vi "Read ADU Packet1.vi"(8 "error in":errorcluster, 10 "isMaster (f)":bool, 11 "RTU transmission data unit in":refnum<class "RTU Data Unit.lvclass">) -> (0 "error out":errorcluster, 1 "modbus data unit":refnum<class "Modbus Data Unit.lvclass">, 3 "RTU transmission data unit out":refnum<class "RTU Data Unit.lvclass">, 5 "PDU Valid?":bool)   [LabVIEW 2021, in "RTU Data Unit.lvclass"]
doc: "This uses the protocol layer to read a modbus packet off of the bus, wrapped in the RTU transmission data unit."
uses:
  RTU Data Unit.lvclass
  D:/my_projects/projects/Algorithms/Labview/21/Modbus_v121c/Transmission Data Unit/Serial Interface/Serial Data Unit.lvclass
  D:/my_projects/projects/Algorithms/Labview/21/Modbus_v121c/Transmission Data Unit/Transmission Data Unit.lvclass
  Modbus Data Unit/Modbus Data Unit.lvclass
  Transmission Data Unit.lvclass/Transmission Data Unit.ctl
  Serial Interface/Serial Data Unit.lvclass/Serial Data Unit.ctl
  Modbus Data Unit/Modbus Data Unit.lvclass/Modbus Data Unit.ctl
  <vilib>/ErrorRing/Error Ring.xnode
  Serial Interface/Serial Data Unit.lvclass
  Transmission Data Unit.lvclass
  Network Interface/Serial Interface/Serial Shared Components/Serial Shared Components.lvlib
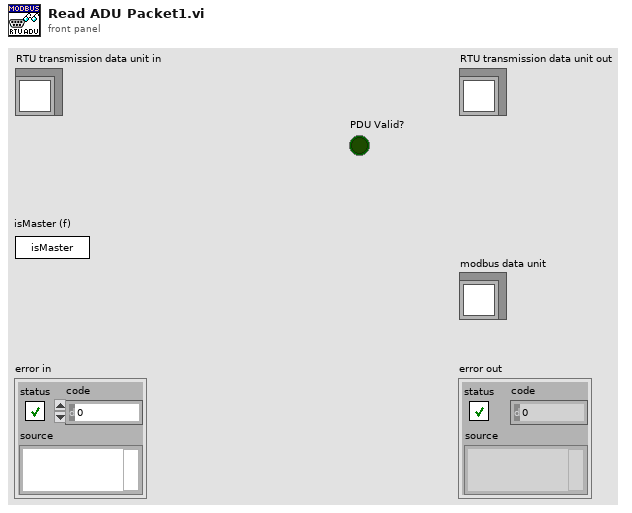
[diagram p1: front panel]
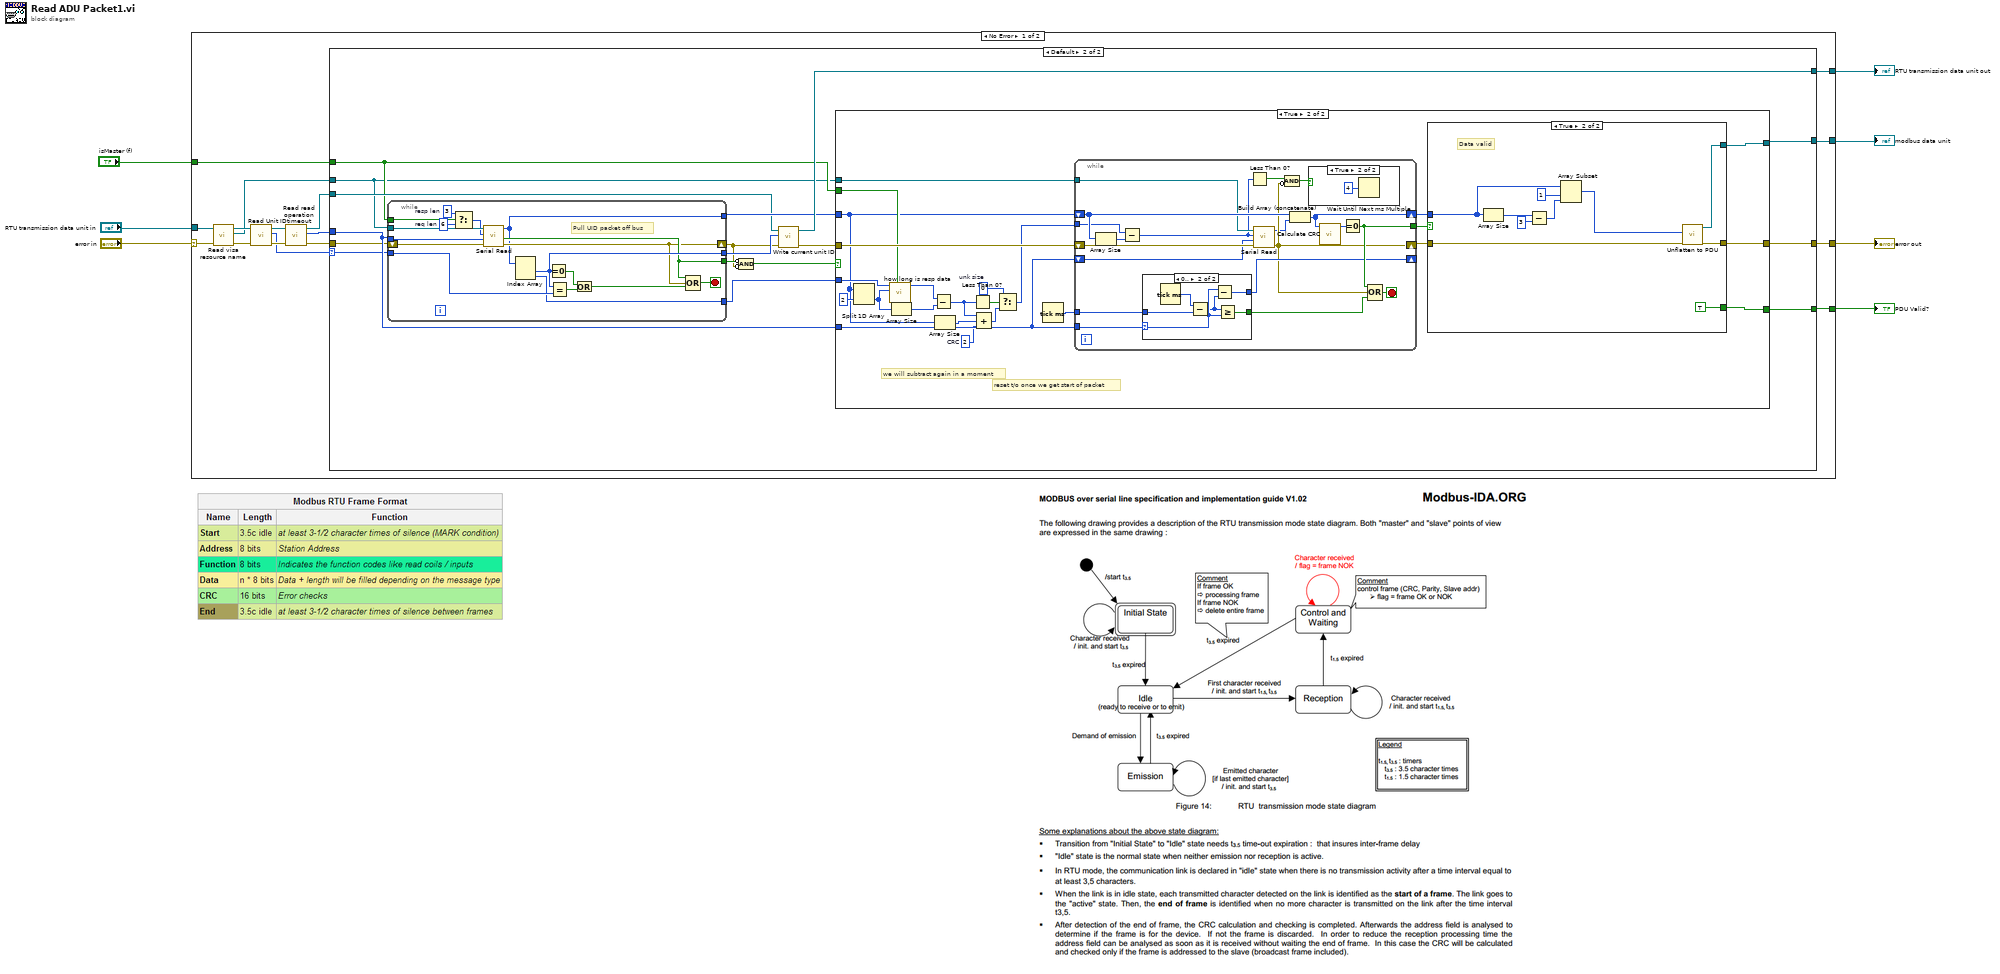
[diagram p0: block diagram]
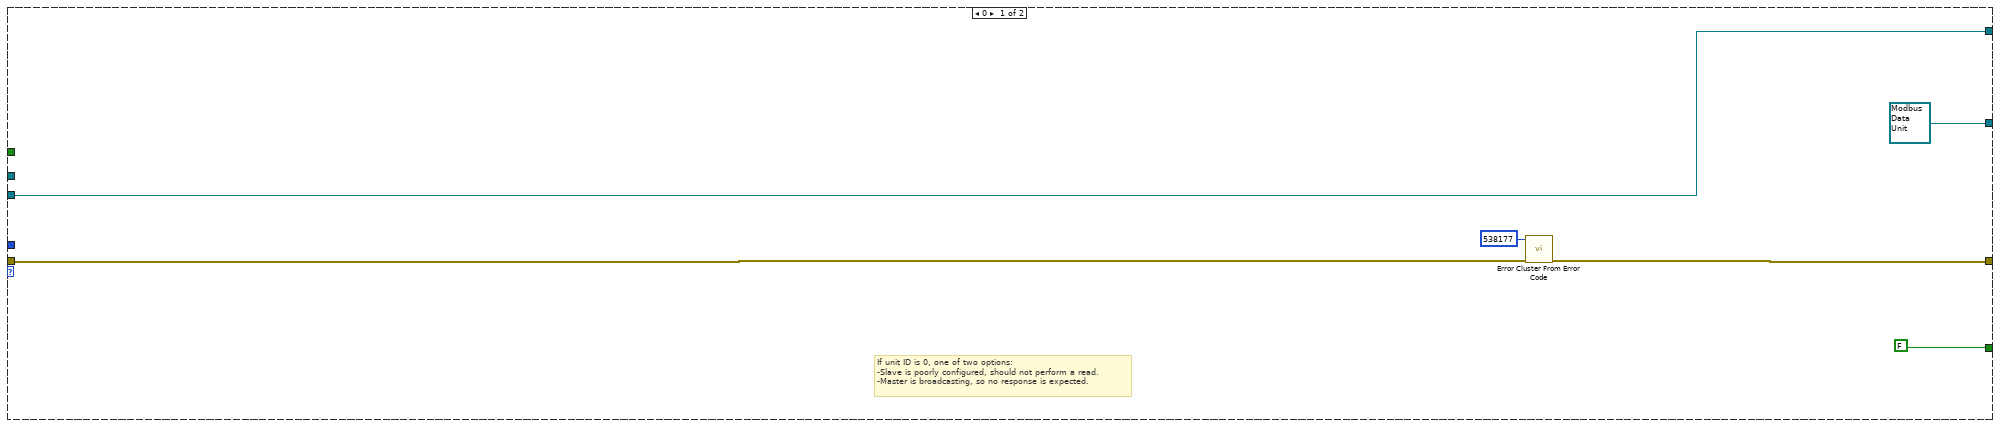
[diagram p2: hidden frame]
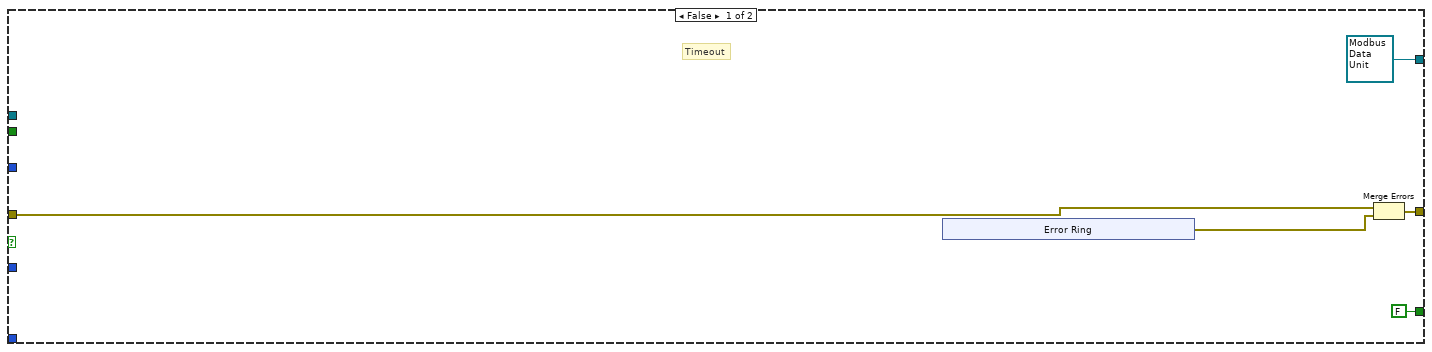
[diagram p3: hidden frame]
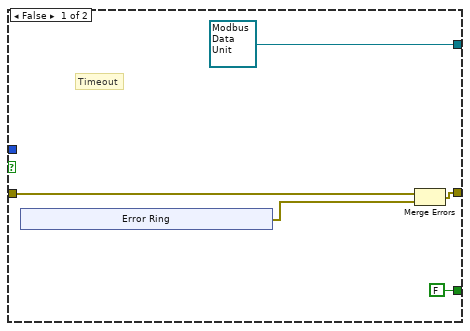
[diagram p4: hidden frame]
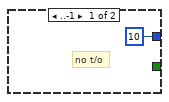
[diagram p6: hidden frame]
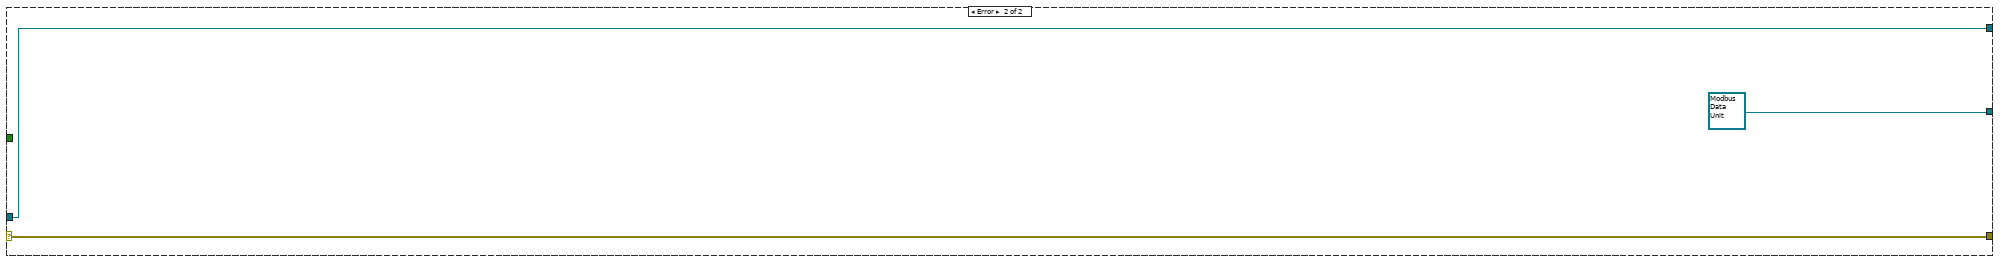
[diagram p7: hidden frame]
diagram:
  n1 = case shown="No Error" "error in" {
    selector: "error in" -> [w9 w145]
    tunnel: [w23 w145] -> w3
    tunnel: "RTU transmission data unit in" -> [w11 w143]
    tunnel: [w22 refnum<class "Modbus Data Unit.lvclass"> refnum ("modbus data unit")] -> w4
    tunnel: [w21 w143] -> w5
    tunnel: [w14 _] -> w2
    tunnel: "isMaster (f)" -> [w13 _]
    frame No Error {
      n2 = call "Read visa resource name.vi"("error in (no error)"=w9, "Serial Data Unit in"=w11) -> ("error out"=w8:errorcluster, "visa resource name"=w10:refnum<visa-resource-name>, "Serial Data Unit out"=w12:refnum<class "RTU Data Unit.lvclass">)  [unwired: 7 in]
      n3 = call "Read Unit ID.vi"("error in"=w8, "transmission data unit in"=w12) -> ("error out"=w18:errorcluster, "unit ID"=w16:u8, "transmission data unit out"=w17:refnum<class "RTU Data Unit.lvclass">)  [unwired: 7 in]
      n4 = call "Read read operation timeout.vi"("error in (no error)"=w18, "transmission data unit in"=w17) -> ("error out"=w19:errorcluster, "read operation timeout"=w15:i32, "transmission data unit out"=w20:refnum<class "RTU Data Unit.lvclass">)  [unwired: 7 in]
      n5 = case shown="Default" w16 {
        selector: w16 -> [_ w43]
        tunnel: w19 -> [w29 w30]
        tunnel: [w25 w46] -> w23
        tunnel: [refnum<class "Modbus Data Unit.lvclass"> refnum ("modbus data unit out") w45] -> w22
        tunnel: w15 -> [_ w44]
        tunnel: w20 -> [w28 w33]
        tunnel: [w28 w42] -> w21
        tunnel: [FALSE w41] -> w14
        tunnel: w13 -> [_ w32]
        tunnel: w10 -> [_ w31]
        frame 0 {
          # "If unit ID is 0, one of two options:\n-Slave is poorly configured, should not perform a read.\n-Master is broadcasting, so no response is expected."
          n6 = call <vilib>:"Error Cluster From Error Code.vi"("error in (no error)"=w29, "error code (0)"=538177) -> ("error out"=w25:errorcluster)  [unwired: 7 in]
        }
        frame Default {
          n7 = while {
            shift-right: [w48] -> w36
            shift-left: w30 -> [w53]
            tunnel: w44 -> [w50]
            tunnel: w43 -> [w59]
            tunnel: [w49] -> w40
            tunnel: [w47] -> w35
            tunnel: w31 -> [w52]
            tunnel: [w58] -> w37
            tunnel: [w57] -> w34
            tunnel: w32 -> [w56]
            stop <- w63 stop-if-true
            w54 = 6  # req len
            w55 = 3  # resp len
            # "Pull UID packet off bus"
            n8 = Select(t=w55, s=w56, f=w54) -> (s? t:f=w51:i32)
            n9 = call "Serial Read.vi"("error in"=w53, "timeout (ms)"=w50, "bytes to read"=w51, "Visa Resource"=w52) -> ("error out"=w48:errorcluster, "timed out?"=w49:bool, "data"=w47:u8[])  [unwired: 5 in]
            n10 = Index Array(array=w47) -> (element #1=w58:u8, element #2=w57:u8)  [unwired: 2 in]
            n11 = Equal To 0?(x=w58) -> (x = 0?=w60:bool)
            n12 = Equal?(x=w58, y=w59) -> (x = y?=w62:bool)
            n13 = Or(x=w60, y=w62) -> (x .or. y?=w61:bool)
            n14 = Compound Arithmetic op=OR(w49, w48, w61) -> (w63:bool)
          }
          n15 = Compound Arithmetic op=AND(invert w40, invert w36) -> (w39:bool)
          n16 = call "Write current unit ID.vi"("error in"=w36, "request unit ID"=w37, "Serial Data Unit in"=w33) -> ("error out"=w38:errorcluster, "Serial Data Unit out"=w42:refnum<class "RTU Data Unit.lvclass">)  [unwired: 7 in]
          n17 = case shown="True" w39 {
            tunnel: w38 -> [w66 w96]
            tunnel: [w67 w90] -> w46
            tunnel: [refnum<class "Modbus Data Unit.lvclass"> refnum ("modbus data unit out") w91] -> w45
            tunnel: w31 -> [_ w94]
            tunnel: w35 -> [_ w74]
            tunnel: w44 -> [_ w82]
            tunnel: [FALSE w88] -> w41
            tunnel: w32 -> [_ w84]
            tunnel: w34 -> [_ w83]
            frame False {
              # "Timeout"
              n18 = xnode "Error Ring"() -> ("error out"=w68:errorcluster)
              n19 = Merge Errors(w66, w68) -> (w67:errorcluster)
            }
            frame True {
              w73 = 2  # CRC
              w80 = 0  # unk size
              # "reset t/o once we get start of packet"
              # "we will subtract again in a moment"
              n20 = Split 1D Array(array=w74, index=2) -> (second subarray=w85:u8[])  [unwired: 1 out]
              n21 = call "how long is resp data.vi"("resp (t) req(f)"=w84, "first (1/4) bytes"=w85, "func"=w83) -> ("bytes in PDU  after func"=w86:i32)  [unwired: 8 in]
              n22 = Array Size(array=w85) -> (size(s)=w87:i32)
              n23 = Subtract(x=w86, y=w87) -> (x-y=w77:i32)
              n24 = Array Size(array=w74) -> (size(s)=w75:i32)
              n25 = Less Than 0?(x=w77) -> (x < 0?=w81:bool)
              n26 = Compound Arithmetic op=ADD(w77, w75, w73) -> (w78:i32)
              n27 = Select(t=w80, s=w81, f=w78) -> (s? t:f=w79:i32)
              n28 = Tick Count (ms)() -> (millisecond timer value=w95:u32)
              n29 = while {
                shift-right: [w119] -> w92
                shift-left: w96 -> [w121]
                tunnel: w95 -> [w134]
                tunnel: w82 -> [w129]
                shift-right: [w131] -> w89
                shift-left: w74 -> [w127]
                tunnel: w94 -> [w118]
                tunnel: [w130] -> w93
                shift-right: [w124] -> _
                shift-left: w82 -> [w120]
                tunnel: w79 -> [w125]
                stop <- w133 stop-if-true
                n30 = Array Size(array=w127) -> (size(s)=w126:i32)
                n31 = Subtract(x=w125, y=w126) -> (x-y=w117:i32)
                n32 = case shown="0.." w129 {
                  selector: w129 -> [_ w139]
                  tunnel: w134 -> [_ w142]
                  tunnel: [_ w140] -> w128
                  tunnel: [u32 10 w137] -> w124
                  frame ..-1 {
                    # "no t/o"
                  }
                  frame 0.. {
                    n33 = Tick Count (ms)() -> (millisecond timer value=w141:u32)
                    n34 = Subtract(x=w141, y=w142) -> (x-y=w138:u32)
                    n35 = Subtract(x=w139, y=w138) -> (x-y=w137:u32)
                    n36 = Greater Or Equal?(x=w138, y=w139) -> (x >= y?=w140:bool)
                  }
                }
                n37 = Less Than 0?(x=w117) -> (x < 0?=w122:bool)
                n38 = call "Serial Read.vi"("error in"=w121, "timeout (ms)"=w120, "bytes to read"=w117, "Visa Resource"=w118) -> ("error out"=w119:errorcluster, "data"=w116:u8[])  [unwired: 5 in, 1 out]
                n39 = Compound Arithmetic op=AND(w122, invert w119) -> (w123:bool)
                n40 = Build Array (concatenate)(w127, w116) -> (w131:u8[])
                n41 = case shown="True" w123 {
                  frame False {
                  }
                  frame True {
                    n42 = Wait Until Next ms Multiple(millisecond multiple=u32 4) -> ()  [unwired: 1 out]
                  }
                }
                n43 = call "Calculate CRC.vi"("data"=w131) -> ("CRC-16"=w132:u16)  [unwired: 10 in]
                n44 = Equal To 0?(x=w132) -> (x = 0?=w130:bool)
                n45 = Compound Arithmetic op=OR(w130, w119, w128) -> (w133:bool)
              }
              n46 = case shown="True" w93 {
                tunnel: w92 -> [w99 w113]
                tunnel: [refnum<class "Modbus Data Unit.lvclass"> refnum ("modbus data unit") w114] -> w91
                tunnel: [w98 w115] -> w90
                tunnel: w89 -> [_ w107]
                tunnel: [FALSE TRUE] -> w88
                frame False {
                  # "Timeout"
                  n47 = xnode "Error Ring"() -> ("error out"=w100:errorcluster)
                  n48 = Merge Errors(w99, w100) -> (w98:errorcluster)
                }
                frame True {
                  # "Data valid"
                  n49 = Array Size(array=w107) -> (size(s)=w111:i32)
                  n50 = Subtract(x=w111, y=3) -> (x-y=w109:i32)
                  n51 = Array Subset(array=w107, index=1, length=w109) -> (w108:u8[])
                  n52 = call "Unflatten to PDU.vi"("error in"=w113, "modbus data unit data"=w108) -> ("error out"=w115:errorcluster, "modbus data unit out"=w114:refnum<class "Modbus Data Unit.lvclass">)  [unwired: 8 in]
                }
              }
            }
          }
        }
      }
    }
    frame Error {
    }
  }
  "RTU transmission data unit out" <- w5
  "modbus data unit" <- w4
  "error out" <- w3
  "PDU Valid?" <- w2
